vi "Render Model.Tester.vi"() -> ()   [LabVIEW 2017, in "PendulumLoop.lvlib"]
uses:
  PendulumLoop.lvlib
  Render Model.PendulumData.ctl
panel:
  in  "Reset Camera":bool
  out "3D Picture":refnum<vi>(3d-picture)
  in  "Cart X":sgl
  in  "Pendulum Render":T1={"Angle"=0.0, "Lenght"=50.0, "X"=0.0, "Y"=25.0}
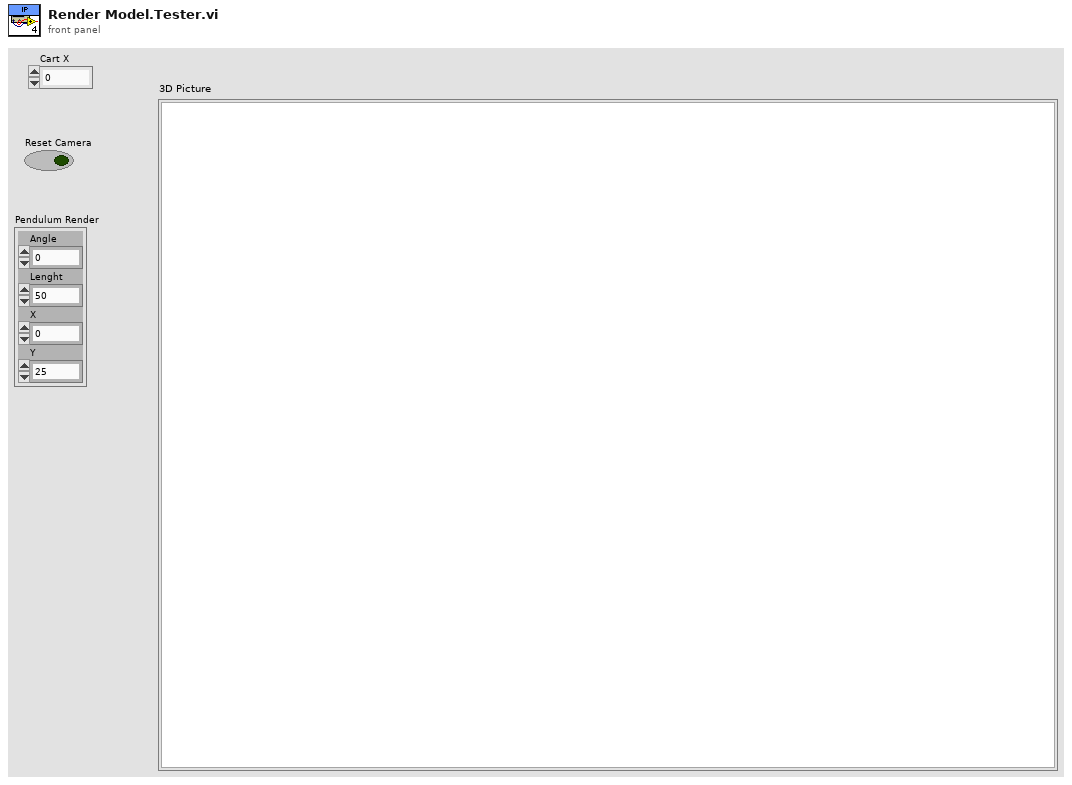
[diagram p1: front panel]
types:
  T1 = typedef "PendulumLoop.lvlib/Render Model.PendulumData.ctl" = cluster{"Angle":sgl, "Lenght":sgl, "X":sgl, "Y":sgl}
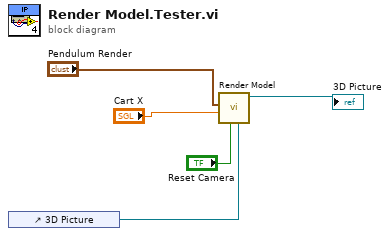
[diagram p0: block diagram]
diagram:
  n1 = control-ref of="3D Picture"() -> (w2:refnum<vi>)
  n2 = call "Render Model.vi"("3D Picture 2"=w2, "Reset Camera"="Reset Camera", "Cart X"="Cart X", 10:"Pendulum Render") -> ("Scene Object Out"=→"3D Picture":refnum<vi>)  [unwired: 7 in]
